vi "subMatchFirstFromPatterns.vi"(9 "patterns":string[](array[string]), 10 "exact match?":bool, 11 "string in":string) -> (1 "index":i32, 2 "matched string":string, 3 "found?":bool)   [LabVIEW 2020, in "CommonHelpers.lvlib"]
uses:
  CommonHelpers.lvlib
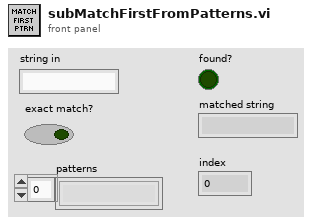
[diagram p1: front panel]
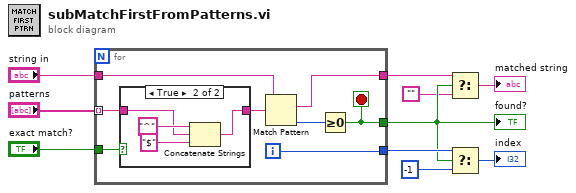
[diagram p0: block diagram]
diagram:
  n1 = for {
    tunnel: "patterns" -> [w12] mode=indexing
    tunnel: [w17] -> w5
    tunnel: "string in" -> [w16]
    tunnel: [w15] -> w8
    tunnel: [w14] -> w4
    tunnel: "exact match?" -> [w11]
    i -> [w15]
    stop <- w17 stop-if-true
    n2 = case shown="True" w11 {
      tunnel: [w19 w21] -> w13
      tunnel: w12 -> [w19 w20]
      frame False {
      }
      frame True {
        n3 = Concatenate Strings("^" ("string"), w20, "$" ("string")) -> (w21:string)
      }
    }
    n4 = Match Pattern(string=w16, regular expression=w13) -> (match substring=w14:string, offset past match=w18:i32)  [unwired: 1 in, 2 out]
    n5 = Greater Or Equal To 0?(x=w18) -> (x >= 0?=w17:bool)
  }
  "found?" <- w5
  n6 = Select(t=w4, s=w5, f="") -> (s? t:f=→"matched string":string)
  n7 = Select(t=w8, s=w5, f=-1) -> (s? t:f=→"index":i32)
